vi "Error Query.vi"(0 "VISA resource name":refnum<visa-resource-name>, 11 "error in (no error)":errorcluster) -> (4 "VISA resource name out":refnum<visa-resource-name>, 6 "Error Code":i32[](array[numeric]), 8 "Error Message":string, 15 "error out":errorcluster)   [LabVIEW 2020]
doc: "Queries the instrument for any errors in the instrument's error queue. It will continue to read errors until all errors have been read from the instrument. Any errors will be returned in the <B>error out</B> control.\n\n<B>Note:</B>\nThis VI is called automatically by most driver VIs so it is not usually necessary to call this in an application."
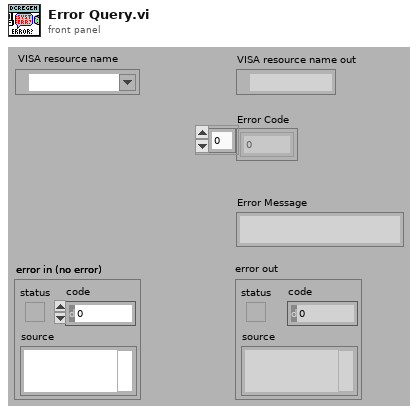
[diagram p1: front panel]
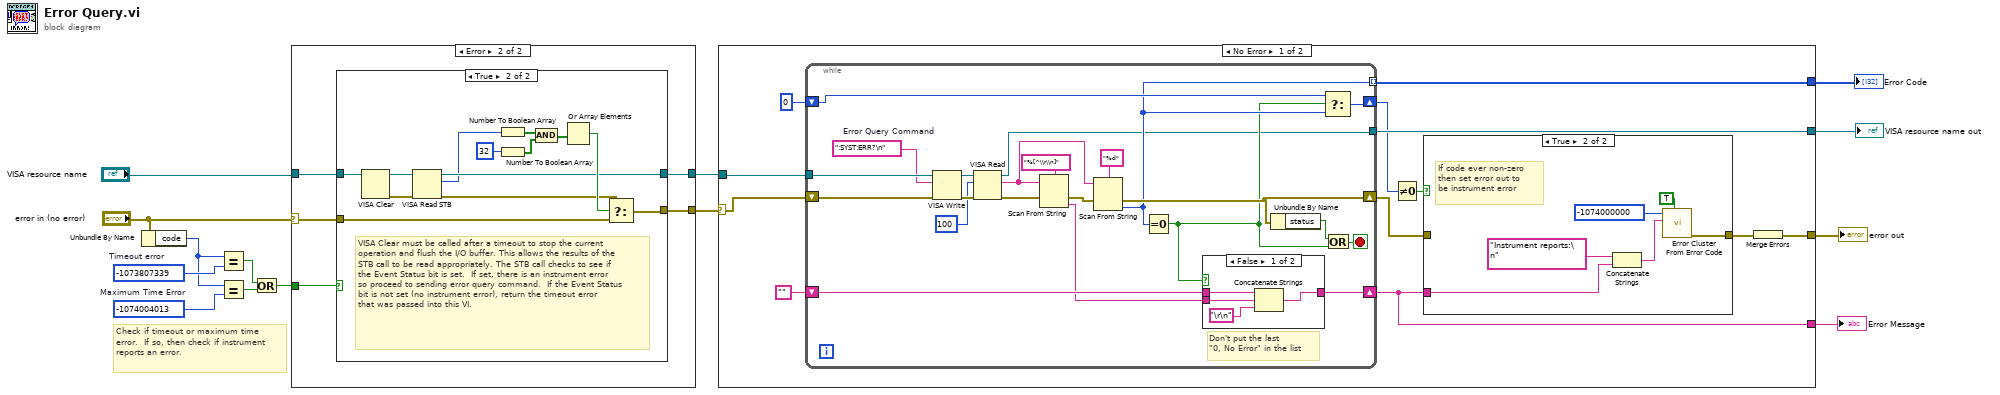
[diagram p0: block diagram]
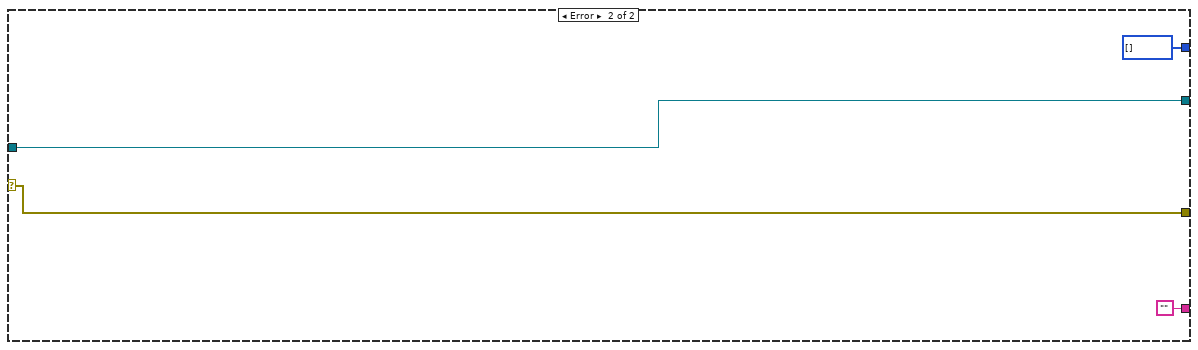
[diagram p4: hidden frame]
diagram:
  w10 = -1074004013  # Maximum Time Error
  w12 = -1073807339  # Timeout error
  # "Check if timeout or maximum time error.  If so, then check if instrument reports an error."
  n1 = Unbundle By Name("error in (no error)") -> ("code"=w11:i32)
  n2 = Equal?(x=w11, y=w12) -> (x = y?=w8:bool)
  n3 = Equal?(x=w11, y=w10) -> (x = y?=w9:bool)
  n4 = Or(x=w8, y=w9) -> (x .or. y?=w7:bool)
  n5 = case shown="Error" "error in (no error)" {
    selector: "error in (no error)" -> [w15 w19]
    tunnel: "VISA resource name" -> [w16 w21]
    tunnel: [w16 w20] -> w13
    tunnel: [w15 w18] -> w14
    tunnel: w7 -> [_ w17]
    frame No Error {
    }
    frame Error {
      n6 = case shown="True" w17 {
        tunnel: w21 -> [w23 w29]
        tunnel: [w23 w26] -> w20
        tunnel: w19 -> [w22 w32]
        tunnel: [w22 w31] -> w18
        frame False {
          # "Error code not a timeout, so best to pass on to user."
        }
        frame True {
          # "VISA Clear must be called after a timeout to stop the current operation and flush the I/O buffer. This allows the results of the  STB call to be read appropriately. The STB call checks to see if the Event Status bit is set.  If set, there is an instrument error so proceed to sending error query command.  If the Event Status bit is not set (no instrument error), return the timeout error that was passed into this VI."
          n7 = VISA Clear(VISA resource name=w29) -> (VISA resource name out=w28:refnum<visa-resource-name>, error out=w27:errorcluster)  [unwired: 1 in]
          n8 = VISA Read STB(8:w27, 11:w28) -> (0:w25:errorcluster, 2:w24:u16, 3:w26:refnum<visa-resource-name>)
          n9 = Number To Boolean Array(number=w24) -> (Boolean array=w33:bool[])
          n10 = Number To Boolean Array(number=32) -> (Boolean array=w35:bool[])
          n11 = And(x=w33, y=w35) -> (x .and. y?=w34:bool[])
          n12 = Or Array Elements(Boolean array=w34) -> (logical OR=w30:bool)
          n13 = Select(t=w25, s=w30, f=w32) -> (s? t:f=w31:errorcluster)
        }
      }
    }
  }
  n14 = case shown="No Error" w14 {
    selector: w14 -> [w37 w83]
    tunnel: [w48 w86] -> w4
    tunnel: w13 -> [w47 w86]
    tunnel: [w45 w83] -> w3
    tunnel: [w40 ""] -> w2
    tunnel: [w39 i32[] []] -> w1
    frame No Error {
      n15 = while {
        tunnel: [w58] -> w48
        tunnel: w47 -> [w63]
        shift-right: [w72] -> w40
        shift-left: "" -> [w74]
        shift-right: [w70] -> w41
        shift-left: 0 -> [w71]
        shift-right: [w69] -> w38
        shift-left: w37 -> [w64]
        tunnel: [w66] -> w39 mode=indexing
        stop <- w76 stop-if-true
        w62 = ":SYST:ERR?\n"  # Error Query Command
        # "Don't put the last\n\"0, No Error\" in the list"
        n16 = VISA Write(VISA resource name=w63, write buffer=w62, error in (no error)=w64) -> (VISA resource name out=w60:refnum<visa-resource-name>, error out=w61:errorcluster)  [unwired: 1 out]
        n17 = VISA Read(VISA resource name=w60, byte count=u32 100, error in (no error)=w61) -> (VISA resource name out=w58:refnum<visa-resource-name>, read buffer=w57:string, error out=w59:errorcluster)  [unwired: 1 out]
        n18 = Scan From String(format string="%[^\\r\\n]", input string=w57, error in=w59) -> (error out=w68:errorcluster, output 1=w73:string)  [unwired: 2 in, 2 out]
        n19 = Scan From String(format string="%d", input string=w57, error in=w68) -> (error out=w69:errorcluster, output 1=w66:i32)  [unwired: 2 in, 2 out]
        n20 = Equal To 0?(x=w66) -> (x = 0?=w65:bool)
        n21 = case shown="False" w65 {
          tunnel: w74 -> [w81 w82]
          tunnel: w73 -> [w79 _]
          tunnel: [w78 w82] -> w72
          frame False {
            n22 = Concatenate Strings(w81, w79, "\r\n") -> (w78:string)
          }
          frame True {
          }
        }
        n23 = Unbundle By Name(w69) -> ("status"=w67:bool)
        n24 = Select(t=w71, s=w65, f=w66) -> (s? t:f=w70:i32)
        n25 = Or(x=w67, y=w65) -> (x .or. y?=w76:bool)
      }
      n26 = Not Equal To 0?(x=w41) -> (x != 0?=w43:bool)
      n27 = case shown="True" w43 {
        tunnel: w40 -> [_ w54]
        tunnel: [w49 w50] -> w42
        tunnel: w38 -> [w49 _]
        frame False {
        }
        frame True {
          # "If code ever non-zero\nthen set error out to\nbe instrument error"
          n28 = Concatenate Strings("Instrument reports:\n" ("Source"), w54) -> (w51:string)
          n29 = call "Error Cluster From Error Code.vi"("show call chain? (False)"=TRUE, "error message (\"\")"=w51, "error code (0)"=-1074000000 ("Code")) -> ("error out"=w50:errorcluster)  [unwired: 6 in]
        }
      }
      n30 = Merge Errors(w42) -> (w45:errorcluster)
    }
    frame Error {
    }
  }
  "VISA resource name out" <- w4
  "error out" <- w3
  "Error Message" <- w2
  "Error Code" <- w1
